vi "Write Report Path.vi"(10 "Report Path":path, 11 "Test Report.Default in":refnum<class "Test Report.Template.lvclass">) -> (3 "Test Report.Default out":refnum<class "Test Report.Template.lvclass">)   [LabVIEW 2013, in "Caraya.lvlib" / "Test Report.Template.lvclass"]
uses:
  Test Report.Template.lvclass
  Test Report.Template.lvclass/Test Report.Template.ctl
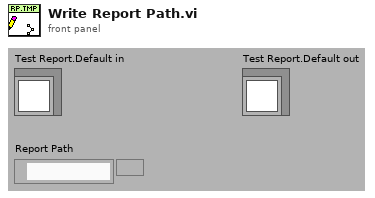
[diagram p1: front panel]
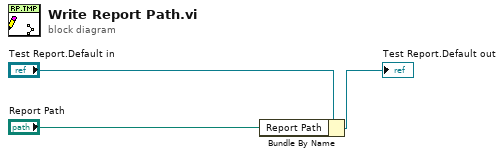
[diagram p0: block diagram]
diagram:
  n1 = Bundle By Name(cluster="Test Report.Default in", "Report Path"="Report Path") -> (→"Test Report.Default out":refnum<class "Test Report.Template.lvclass">)
